vi "Control_Rack_Controler.vi"(0 "Times":dbl[](array[numeric]), 1 "Voltages Toroidal (Keep below |10|)":dbl[](array[numeric]), 2 "Voltages Helical (Keep below |10|)":dbl[](array[numeric]), 3 "error out":errorcluster, 4 "Data out 2":T1) -> (5 "error out 2":errorcluster, 6 "Data out":T1)   [LabVIEW 2017]
uses:
  Type_Defs/Data.ctl
  Type_Defs/Diagnostics.ctl
  Type_Defs/Systems.ctl
  <vilib>/DAQmx/write.llb/DAQmx Write (Analog DBL 1Chan 1Samp).vi
  <vilib>/DAQmx/create/channels.llb/DAQmx Create Channel (AO-Voltage-Basic).vi
  <vilib>/DAQmx/miscellaneous.llb/DAQmx Fill In Error Info.vi
panel:
  out "hel_cur":dynamicdata(graph) caption="Helix Current Feedback"
  out "hel_vol":dynamicdata(graph) caption="Helix Voltage Feedback"
  out "hel_cur_set":dynamicdata(graph) caption="Helix Limited Current Set Point"
  out "torr_cur_set":dynamicdata(graph) caption="Torroidal Limited Current Set Point"
  out "torr_vol":dynamicdata(graph) caption="Torroidal Voltage Feedback"
  out "torr_cur":dynamicdata(graph) caption="Torroidal Current Feedback"
  out "Voltage Toroidal":dbl
  out "Time":dbl
  out "Voltage Helical":dbl
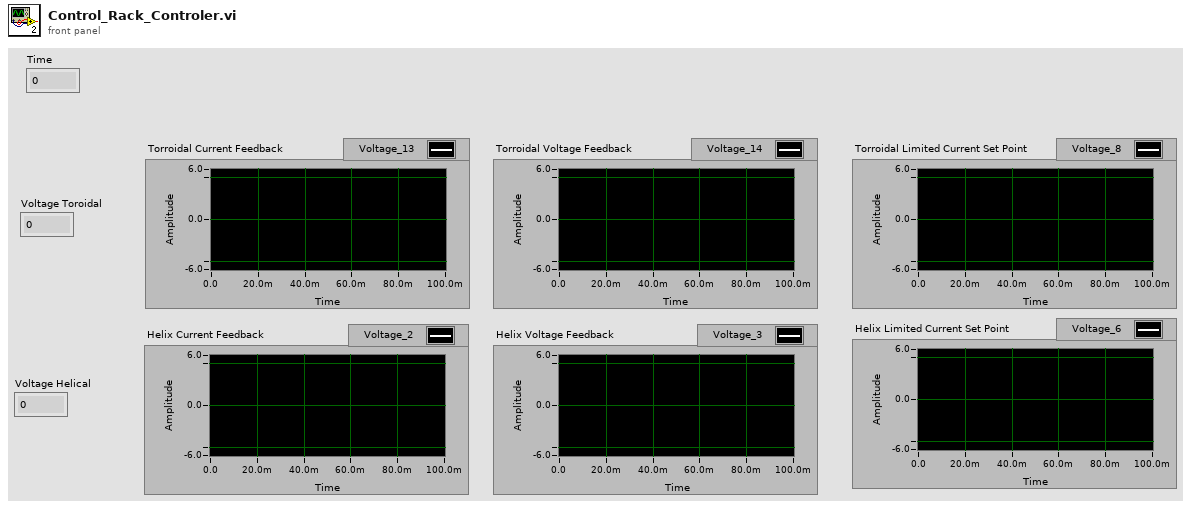
[diagram p1: front panel]
types:
  T1 = typedef "Data.ctl" = cluster{"User Name":string, "Experiment Number":i32, "Start Time":timestamp, "Data":dbl[], "Step Number":i32, "Step Instructions":string, "Diagnostics":T2, "Experiment Purpose":string, "Experiment State":enum16{"Off", "Setting Up", "Ready", "In Progress", "Shutting Down"}, "Systems":T3, "Vacuum Pressure":dbl, "Fieldpoints":cluster{"System Boolean Fieldpoints":cluster{"Compressed Air":refnum<k21>, "T-20kV Power Switch":refnum<k21>, "T-Rectifier":refnum<k21>, "Engage Interlock":refnum<k21>, "Ventilator":refnum<k21>, "Magnetron":refnum<k21>, "H-20kV Power Switch":refnum<k21>, "H-Rectifier":refnum<k21>, "Main Water Pump":refnum<k21>, "WEGA Water Pump":refnum<k21>, "Gas Inlet Valves":refnum<k21>}, "Step Fieldpoints":cluster{"Exhaust Ventillator":refnum<k21>, "Compressed Air":refnum<k21>, "Water Pressure":refnum<k21>, "Interlock":refnum<k21>, "Toroidal Power Supply 1":refnum<k21>, "Toroidal Power Supply 2":refnum<k21>, "Toroidal Rectifier":refnum<k21>, "Helical Power Supply":refnum<k21>, "Helical Rectifier":refnum<k21>, "6kW Magnetron Standby":refnum<k21>, "20kW Magnetron Standby":refnum<k21>}}, "Pressure History":cluster{"Seconds into Experiment":i32[], "Pressure Data":dbl[]}, "Time Computer Control":dbl[], "Toroidal Voltage Computer Control":dbl[], "Helical Voltage Computer Control":dbl[], "Toroidal Current":dbl[], "Toroidal Voltage":dbl[], "Toroidal Current Set Point":dbl[], "Helical Current Set Point":dbl[], "Helical Voltage":dbl[], "Helical Current":dbl[]}
  T2 = typedef "Diagnostics.ctl" = cluster{"Langmuir Probe":bool, "Rogowski 1":bool, "Rogowski 2":bool, "Rogowski 3":bool, "B-dot 1":bool, "B-dot 2":bool}
  T3 = typedef "Systems.ctl" = cluster{"Compressed Air":bool, "T-20kV Power Switch":bool, "T-Rectifier":bool, "Engage Interlock":bool, "Ventilator":bool, "Magnetron":bool, "H-20kV Power Switch":bool, "H-Rectifier":bool, "Main Water Pump":bool, "WEGA Water Pump":bool, "Gas Inlet Valves":bool}
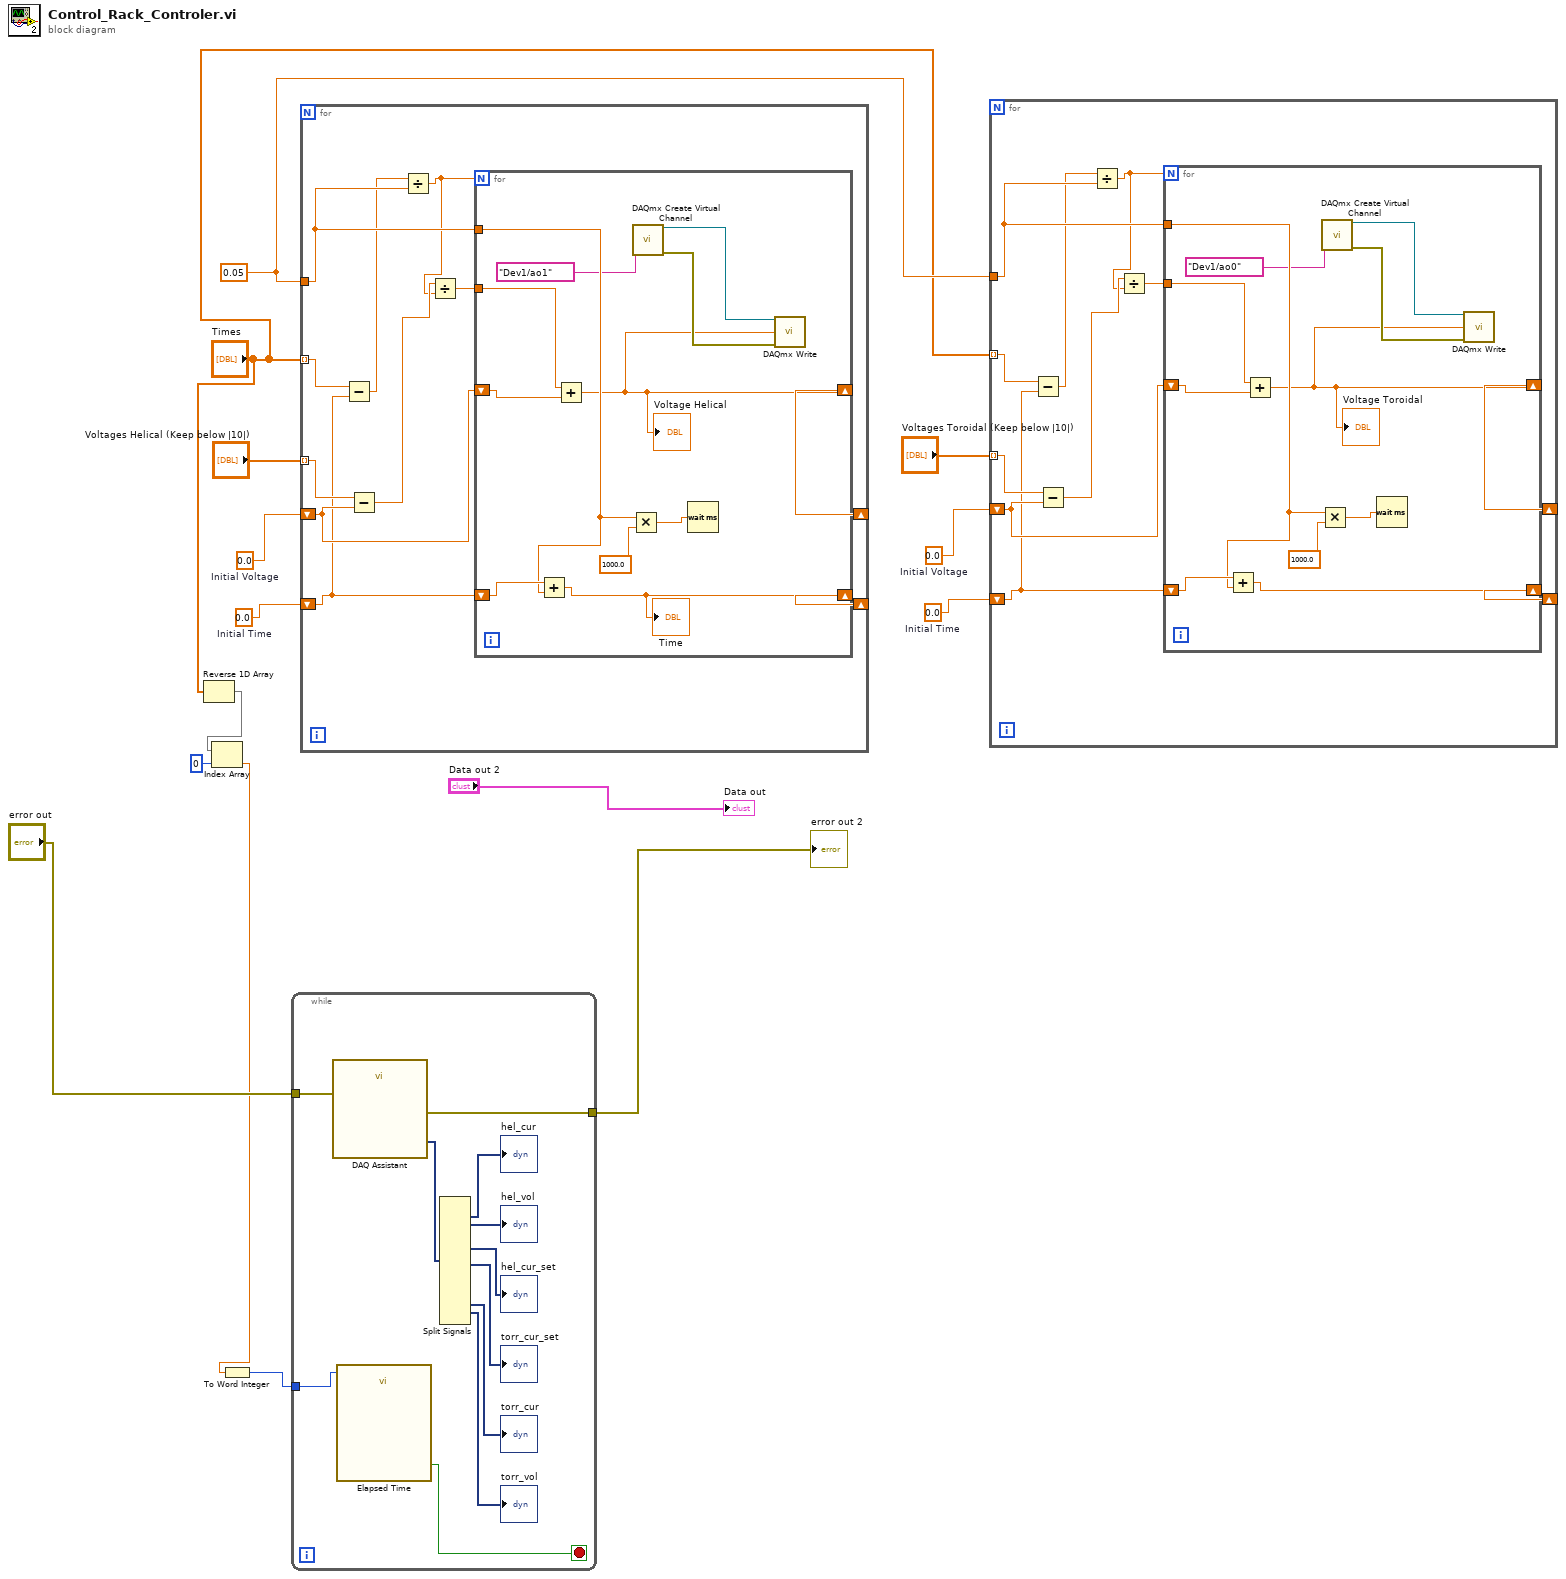
[diagram p0: block diagram]
diagram:
  w9 = 0.05 ("Timestep (in seconds, keep above 1/20s)")
  w12 = 0.0  # Initial Time
  w11 = 0.0  # Initial Voltage
  w13 = 0.0  # Initial Time
  w14 = 0.0  # Initial Voltage
  n1 = Reverse 1D Array(array="Times") -> (reversed array=w7:dbl[])
  n2 = Index Array(array=w7, index=0) -> (element=w2:dbl)
  n3 = To Word Integer(number=w2) -> (16bit integer=w1:i16)
  n4 = while {
    tunnel: "error out" -> [w19]
    tunnel: [w18] -> w3
    tunnel: w1 -> [w16]
    stop <- w17 stop-if-true
    n5 = call "DAQ Assistant"("error in"=w19) -> ("data"=w25:dynamicdata, "error out"=w18:errorcluster)  [unwired: 16 in, 1 out]
    n6 = call "Elapsed Time"("Time Target (s)"=w16) -> ("Time has Elapsed"=w17:bool)  [unwired: 11 in, 7 out]
    n7 = Split Signals(w25) -> (→"hel_cur":dynamicdata, →"hel_vol":dynamicdata, →"hel_cur_set":dynamicdata, →"torr_cur_set":dynamicdata, →"torr_cur":dynamicdata, →"torr_vol":dynamicdata)  [unwired: 16 in, 10 out]
  }
  "error out 2" <- w3
  n8 = for {
    tunnel: "Voltages Helical (Keep below |10|)" -> [w37] mode=indexing
    tunnel: "Times" -> [w30] mode=indexing
    tunnel: w9 -> [w32]
    shift-right: [w33] -> _
    shift-left: w14 -> [w36]
    shift-right: [w31] -> _
    shift-left: w13 -> [w29]
    n9 = Subtract(x=w30, y=w29) -> (x-y=w28:dbl)
    n10 = Subtract(x=w37, y=w36) -> (x-y=w35:dbl)
    n11 = Divide(x=w28, y=w32) -> (x/y=w27:dbl)
    n12 = Divide(x=w35, y=w27) -> (x/y=w34:dbl)
    n13 = for {
      N: w27 -> [_]
      shift-right: [w38] -> w33
      shift-left: w36 -> [w48]
      tunnel: w34 -> [w47]
      tunnel: w32 -> [w44]
      shift-right: [w42] -> w31
      shift-left: w29 -> [w46]
      n14 = Add(x=w46, y=w44) -> (x+y=w42:dbl)
      "Time" <- w42
      n15 = Add(x=w47, y=w48) -> (x+y=w38:dbl)
      "Voltage Helical" <- w38
      n16 = Multiply(x=w44, y=1000.0) -> (x*y=w45:dbl)
      n17 = call-poly <vilib>:"DAQmx Create Virtual Channel.vi"("physical channels"=tag "Dev1/ao1" ("write channel (torr = ao0, hel = ao1)")) -> ("task out"=w39:refnum<k21>, "error out"=w40:errorcluster)  [unwired: 13 in]
      n18 = Wait (ms)(milliseconds to wait=w45) -> ()  [unwired: 1 out]
      n19 = call-poly <vilib>:"DAQmx Write.vi"("task/channels in"=w39, "data"=w38, "error in"=w40) -> ()  [unwired: 10 in, 3 out]
    }
  }
  n20 = for {
    tunnel: "Voltages Toroidal (Keep below |10|)" -> [w59] mode=indexing
    tunnel: "Times" -> [w52] mode=indexing
    tunnel: w9 -> [w54]
    shift-right: [w55] -> _
    shift-left: w11 -> [w58]
    shift-right: [w53] -> _
    shift-left: w12 -> [w51]
    n21 = Subtract(x=w52, y=w51) -> (x-y=w50:dbl)
    n22 = Subtract(x=w59, y=w58) -> (x-y=w57:dbl)
    n23 = Divide(x=w50, y=w54) -> (x/y=w49:dbl)
    n24 = Divide(x=w57, y=w49) -> (x/y=w56:dbl)
    n25 = for {
      N: w49 -> [_]
      shift-right: [w60] -> w55
      shift-left: w58 -> [w70]
      tunnel: w56 -> [w69]
      tunnel: w54 -> [w66]
      shift-right: [w64] -> w53
      shift-left: w51 -> [w68]
      n26 = Add(x=w68, y=w66) -> (x+y=w64:dbl)
      n27 = Add(x=w69, y=w70) -> (x+y=w60:dbl)
      "Voltage Toroidal" <- w60
      n28 = Multiply(x=w66, y=1000.0) -> (x*y=w67:dbl)
      n29 = call-poly <vilib>:"DAQmx Create Virtual Channel.vi"("physical channels"=tag "Dev1/ao0" ("write channel (torr = ao0, hel = ao1) 2")) -> ("task out"=w61:refnum<k21>, "error out"=w62:errorcluster)  [unwired: 13 in]
      n30 = Wait (ms)(milliseconds to wait=w67) -> ()  [unwired: 1 out]
      n31 = call-poly <vilib>:"DAQmx Write.vi"("task/channels in"=w61, "data"=w60, "error in"=w62) -> ()  [unwired: 10 in, 3 out]
    }
  }
  "Data out" <- "Data out 2"
